vi "Victor Motor Control.vi"(10 "Motor Speed":dbl, 11 "PWM Channel":T1) -> ()   [LabVIEW 2016, in "navX Library.lvlib"]
uses:
  <vilib>/Rock Robotics/SystemInterfaces/DIO/FPGA_DIOPWMChannel.ctl
  <vilib>/Rock Robotics/WPI/SafetyOutput/WPI_SafetyOutputConfigMenu.ctl
  <vilib>/Rock Robotics/WPI/MotorControl/WPI_MotorControlOpen Victor.vi
  navX Library.lvlib
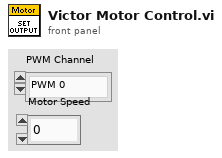
[diagram p1: front panel]
types:
  T1 = typedef "FPGA_DIOPWMChannel.ctl" = enum8{"PWM 0", "PWM 1", "PWM 2", "PWM 3", "PWM 4", "PWM 5", "PWM 6", "PWM 7", "PWM 8", "PWM 9", "PWM MXP 0", "PWM MXP 1", "PWM MXP 2", "PWM MXP 3", "PWM MXP 4", "PWM MXP 5", "PWM MXP 6", "PWM MXP 7", "PWM MXP 8", "PWM MXP 9", "Invalid"}
  T2 = typedef "WPI_SafetyOutputConfigMenu.ctl" = enum16{"Enable", "Disable"}
  T3 = typedef "WPI_MotorControlDeviceRef.ctl" = cluster{"DeviceStatus":errorcluster, "Type":T4, "PWM":cluster{"PWM Channel":T1, "DeadBand":T5}, "CAN":cluster{"Device Number":u8, "SetOutput VI Ref":variant, "GetOutput VI Ref":variant, "Enable VI Ref":variant, "Disable VI Ref":variant, "Data":variant}, "Invert":bool}
  T4 = typedef "WPI_MotorControlType.ctl" = enum16{"PWM", "CAN"}
  T5 = typedef "WPI_PWMDeadband.ctl" = cluster{"Name":string, "maxPositivePwm":i32, "minPositivePwm":i32, "centerPwm":i32, "maxNegativePwm":i32, "minNegativePwm":i32, "angularRange":u16}
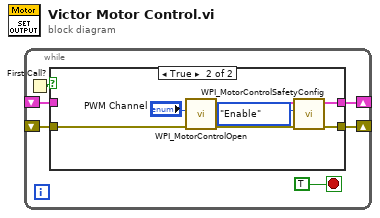
[diagram p0: block diagram]
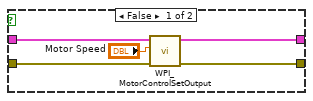
[diagram p2: hidden frame]
diagram:
  n1 = while {
    shift-right: [w1] -> _
    shift-left: _ -> [w4]
    shift-right: [w3] -> _
    shift-left: _ -> [w2]
    stop <- TRUE stop-if-true
    n2 = First Call?() -> (First Call?: T/F=w5:bool)
    n3 = case shown="True" w5 {
      tunnel: w4 -> [w9 w18]
      tunnel: [w10 w15] -> w3
      tunnel: w2 -> [w11 _]
      tunnel: [w8 w13] -> w1
      frame False {
        n4 = call <vilib>:"WPI_MotorControlSetOutput.vi"("error in (no error)"=w9, "Output"="Motor Speed", "MotorControlDevRef"=w11) -> ("error out"=w8:errorcluster, "MotorControlDevRef"=w10:T3)  [unwired: 6 in, 1 out]
      }
      frame True {
        n5 = call-poly <vilib>:"WPI_MotorControlOpen.vi"("error in (no error)"=w18, "PWM Channel"="PWM Channel") -> ("error out"=w14:errorcluster, "MotorControlDeviceRef"=w16:T3)  [unwired: 8 in]
        n6 = call <vilib>:"WPI_MotorControlSafetyConfig.vi"("error in (no error)"=w14, "mode"=WPI_SafetyOutputConfigMenu."Enable", "MotorControlDevRef"=w16) -> ("error out"=w13:errorcluster, "MotorControlDevRef"=w15:T3)  [unwired: 7 in]
      }
    }
  }
